vi "Register Enum Metadata.vi"(8 "error in":errorcluster, 10 "Enum Metadata":T2[](array[typedef]), 11 "gRPCid in":T1) -> (0 "error out":errorcluster, 3 "gRPCid out":T1)   [LabVIEW 2019, in "grpc-lvsupport.lvlib"]
uses:
  grpc-lvsupport.lvlib
  typeDefs/Enum Metadata.ctl
  Shared/grpcId.ctl
  <vilib>/Utility/error.llb/Error Cluster From Error Code.vi
  <vilib>/Utility/error.llb/Simple Error Handler.vi
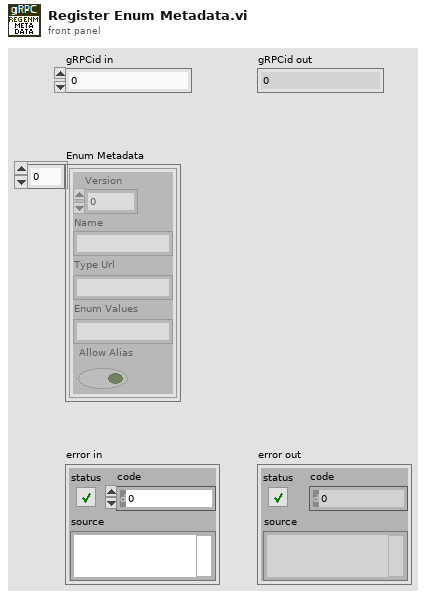
[diagram p1: front panel]
types:
  T1 = typedef "grpc-lvsupport.lvlib/grpcId.ctl" = u64
  T2 = typedef "grpc-lvsupport.lvlib/Enum Metadata.ctl" = cluster{"Version":i32, "Name":string, "Type Url":string, "Enum Values":string, "Allow Alias":bool}
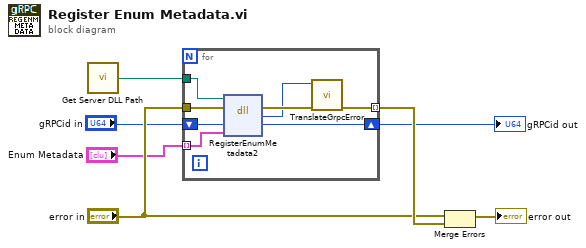
[diagram p0: block diagram]
diagram:
  n1 = call "Get Server DLL Path.vi"() -> ("Server dll path"=w6:path)
  n2 = for {
    tunnel: "Enum Metadata" -> [w13] mode=indexing
    tunnel: "error in" -> [w15]
    tunnel: [w9] -> w7 mode=indexing
    tunnel: w6 -> [w10]
    shift-right: [w11] -> w1
    shift-left: "gRPCid in" -> [w12]
    n3 = dll-call lib="C:/Source/grpc-labview/build/Debug/labview_grpc_server.dll" fn="RegisterEnumMetadata2"(path in=w10, error in=w15, "serverId"=w12, "metadata"=w13) -> (error out=w14:errorcluster, "return type"=w8:i32, "serverId"=w11:T1)  [unwired: 2 in, 1 out]
    n4 = call "TranslateGrpcError.vi"("error in"=w14, "Error Code"=w8) -> ("error out"=w9:errorcluster)  [unwired: 9 in]
  }
  "gRPCid out" <- w1
  n5 = Merge Errors("error in", w7) -> (→"error out":errorcluster)
